vi "TreeRow2String.vi"(8 "类型":enum16{"动作", "组"}(ring), 10 "索引":i32, 11 "TreeControl输入":refnum<vi>) -> (2 "键值串":string, 3 "TreeControl输出":refnum<vi>)   [LabVIEW 2020, in "Curve Editor.lvlib"]
uses:
  Curve Editor.lvlib
  Key Value/Key Value.lvlib
panel:
  # "按类型将树行列表中指定行的数据转换为键值串，并返回这个键值串"
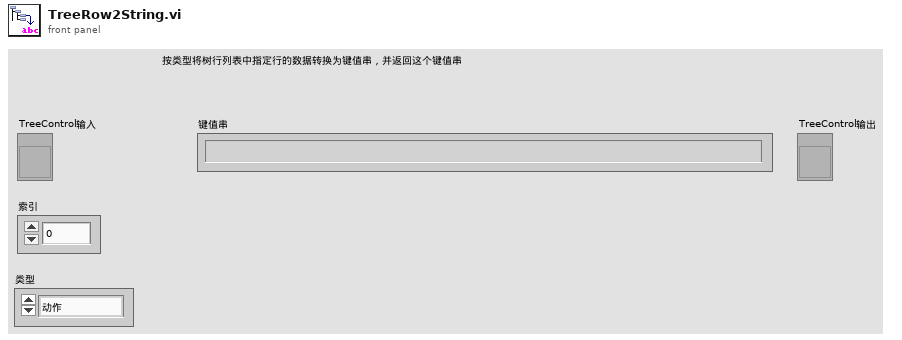
[diagram p1: front panel]
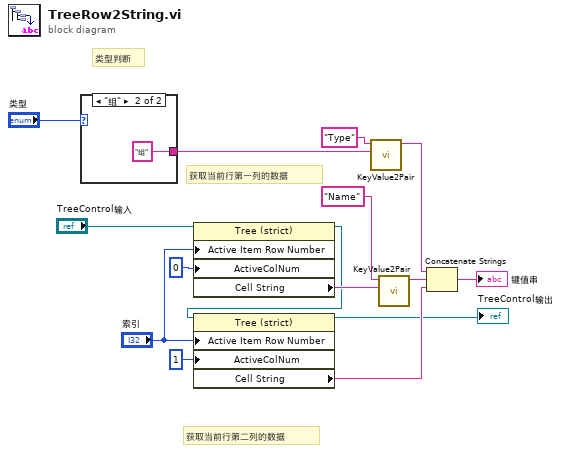
[diagram p0: block diagram]
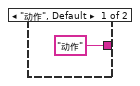
[diagram p2: hidden frame]
diagram:
  # "获取当前行第二列的数据"
  # "获取当前行第一列的数据"
  # "类型判断"
  n1 = case shown="\"组\"" "类型" {
    tunnel: ["动作" ("值") "组" ("值")] -> w6
    frame "动作", Default {
    }
    frame "组" {
    }
  }
  n2 = property class="Tree (strict)"(reference="TreeControl输入", "Active Item Row Number"="索引", "ActiveColNum"=0 ("活动单元格:活动列数")) -> (reference out=w2:refnum<vi>, "Cell String"=w10:string)  [unwired: 1 in, 1 out]
  n3 = property class="Tree (strict)"(reference=w2, "Active Item Row Number"="索引", "ActiveColNum"=1 ("活动单元格:活动列数")) -> (reference out=→"TreeControl输出":refnum<vi>, "Cell String"=w15:string)  [unwired: 1 in, 1 out]
  n4 = call "KeyValue2Pair.vi"("值"=w6, "键"="Type") -> ("键值对"=w13:string)  [unwired: 9 in]
  n5 = call "KeyValue2Pair.vi"("值"=w10, "键"="Name") -> ("键值对"=w14:string)  [unwired: 9 in]
  n6 = Concatenate Strings(w13, w14, w15) -> (→"键值串":string)
